vi "connect.vi"(8 "error in":errorcluster, 11 "API Token":string) -> (0 "error out":errorcluster, 3 "Nominal Client":refnum<class "Nominal Client.lvclass">)   [LabVIEW 2024, in "nominal labview client.lvlib"]
uses:
  nominal labview client.lvlib
  <vilib>/Nominal/Nominal IO Client/Nominal Client/Nominal Client.lvclass
  <vilib>/Nominal/Nominal IO Client/Nominal Client/Nominal Client.lvclass/Nominal Client.ctl
  30398a5e-1de0-42c8-a146-df9120ea344a.vi
  <vilib>/Nominal/Nominal IO Client/Nominal Client/private_data.set.vi
  <vilib>/Utility/file.llb/Application Directory.vi
  <vilib>/Utility/error.llb/Error Cluster From Error Code.vi
  <vilib>/addons/_JKI.lib/REST Client/classes/REST Client/Create REST Client.vi
  <vilib>/addons/_JKI.lib/REST Client/classes/REST Client/REST Client.lvclass
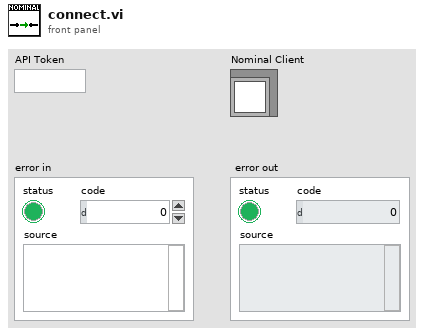
[diagram p1: front panel]
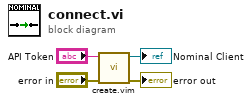
[diagram p0: block diagram]
diagram:
  n1 = call "create.vim"("error in"="error in", "API Token (string or path)"="API Token") -> ("error out"=→"error out":errorcluster, "Nominal Client"=→"Nominal Client":refnum<class "Nominal Client.lvclass">)  [unwired: 8 in]
